vi "fgt detect.vi"(8 "error in (no error)":errorcluster) -> (0 "error out":errorcluster, 2 "type out":T1[](array[typedef]), 3 "SN out":u16[](array[numeric]))   [LabVIEW 2016, in "fgt_SDK.lvlib"]
doc: "Detects all connected Fluigent instrument(s), return their serial number and type"
uses:
  fgt_SDK.lvlib
  TypeDefs/fgt_INSTRUMENT_TYPE.ctl
  dlls/fgt_SDK_32.dll
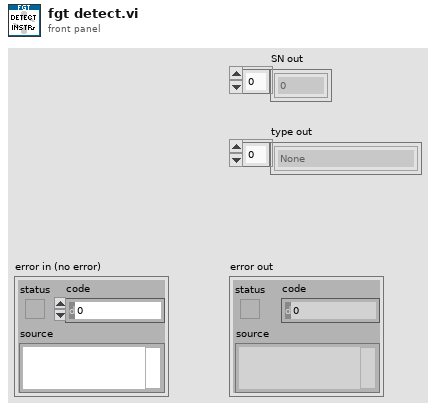
[diagram p1: front panel]
types:
  T1 = typedef "fgt_SDK.lvlib/fgt_INSTRUMENT_TYPE.ctl" = enum32{"None", "MFCS", "MFCS_EZ", "FRP", "LineUP"}
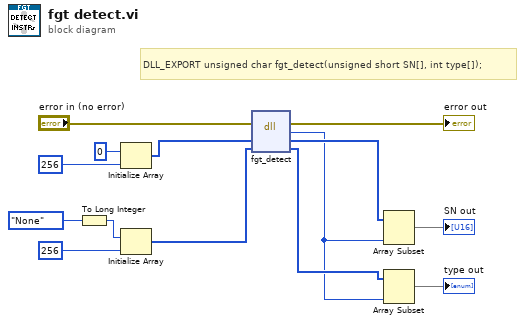
[diagram p0: block diagram]
diagram:
  # "DLL_EXPORT unsigned char fgt_detect(unsigned short SN[], int type[]);"
  n1 = To Long Integer(number=fgt_INSTRUMENT_TYPE."None" ("fgt_INSTRUMENT_TYPE")) -> (32bit integer=w2:i32)
  n2 = Initialize Array(u16 0 ("element"), 256 ("dimension size")) -> (w5:u16[])
  n3 = Initialize Array(w2, 256 ("dimension size")) -> (w4:i32[])
  n4 = dll-call lib="PTH2Zabs D\nMes DocumentsDéveloppementFluigentSDKsfgt-sdk-labviewdllsfgt_SDK_*.*" fn="fgt_detect"(error in="error in (no error)", "SN"=w5, "type"=w4) -> (error out=→"error out":errorcluster, "return type"=w1:u8, "SN"=w12:u16[], "type"=w10:i32[])  [unwired: 2 in, 1 out]
  n5 = Array Subset(array=w12, length=w1) -> (→"SN out":u16[])  [unwired: 1 in]
  n6 = Array Subset(array=w10, length=w1) -> (→"type out":i32[])  [unwired: 1 in]
